vi "GenWave.vi"(2 "Sampling Rate (MHz)":u32=1000, 3 "Start Gap":dbl, 4 "Start Time":dbl, 5 "Offset":dbl min=-1.0 max=1.0 step=0.1 format="%.2p", 6 "T0":dbl, 7 "Wave":T1 {"Phase (Pi)" min=-1.0 max=1.0 step=0.1 format="%.2f"; "Gap (us)" format="%.2f"; "Amplitude" format="%.2f"; "Duration (us)" format="%.2f"; "Frequency (MHz)" format="%.4f"}) -> (0 "End Time":dbl, 1 "Output":i16[](array[numeric]))   [LabVIEW 2014]
uses:
  Wave.ctl
  <vilib>/gmath/NI_Gmath.lvlib
panel:
  in  "Sample Length Unit":u32=32
  in  "Minimal Sample Length":i32=192
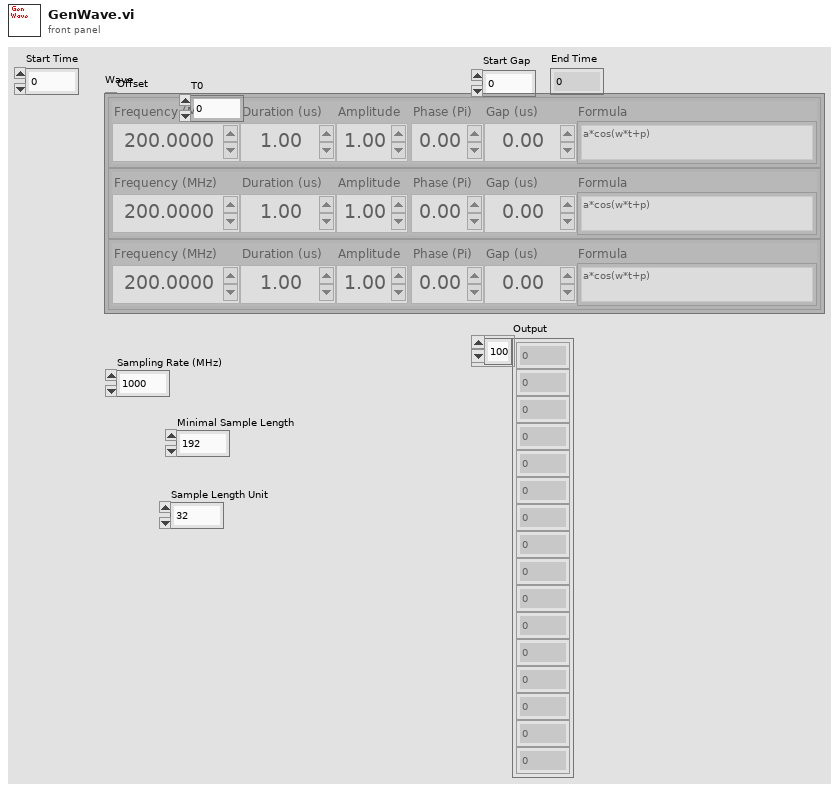
[diagram p1: front panel]
types:
  T1 = typedef "Wave.ctl" = cluster{"Frequency (MHz)":dbl, "Duration (us)":dbl, "Amplitude":dbl, "Phase (Pi)":dbl, "Gap (us)":dbl, "Formula":string}[]
  T2 = cluster{"parameter name":string, "parameter content":string}[]
  T3 = cluster{string, "formula after substitution":string}
  T4 = cluster{"Frequency (MHz)":dbl, "Duration (us)":dbl, "Amplitude":dbl, "Phase (Pi)":dbl, "Gap (us)":dbl, "Formula":string}
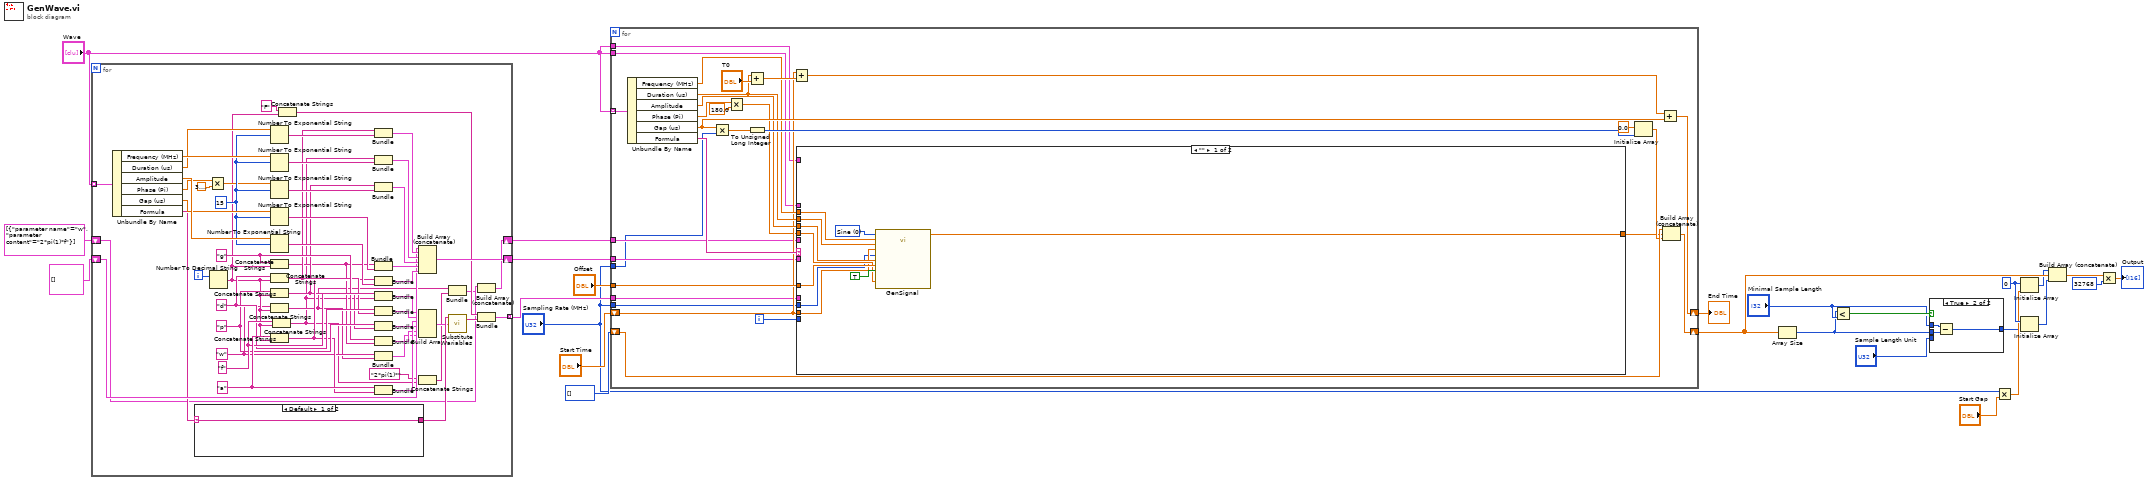
[diagram p0: block diagram]
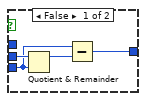
[diagram p2: hidden frame]
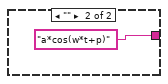
[diagram p3: hidden frame]
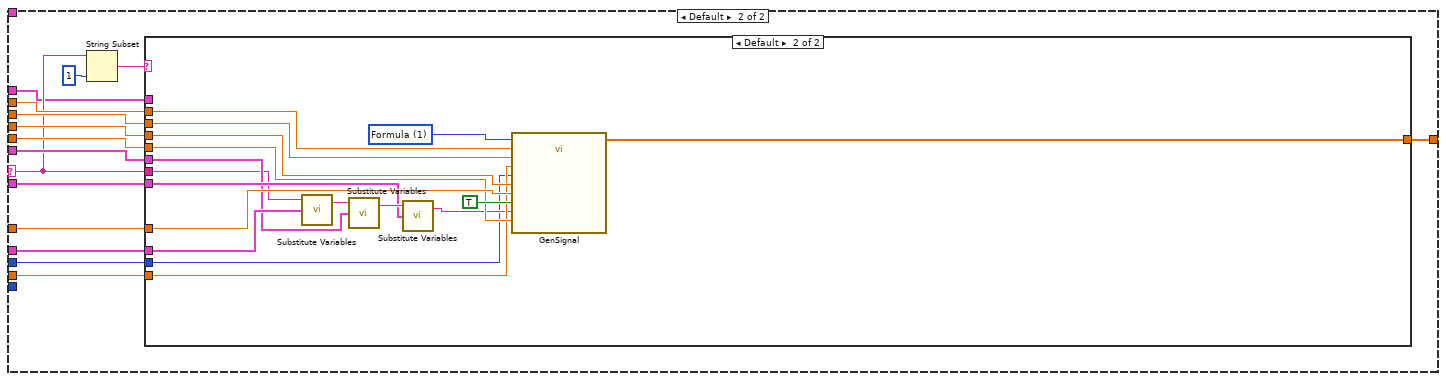
[diagram p4: hidden frame]
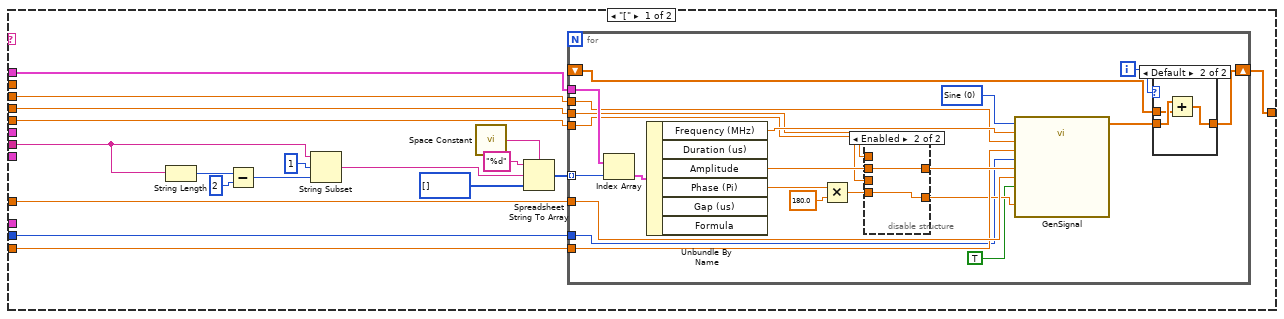
[diagram p5: hidden frame]
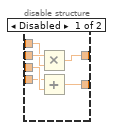
[diagram p6: hidden frame]
diagram:
  w14 = u32 0 ("element")
  n1 = for {
    tunnel: "Wave" -> [w62] mode=indexing
    shift-right: [w63] -> w19
    shift-left: cluster{string, string}[] [] -> [w64]
    tunnel: [w40] -> w18 mode=indexing
    shift-right: [w26] -> w15
    shift-left: T2 [{"parameter name"="w", "parameter content"="2*pi(1)*f"}] ("Substitution Rules") -> [w28]
    i -> [w65]
    w34 = "w" ("string")
    w69 = i16 15 ("width (-)")
    w56 = "a" ("string")
    w54 = "f" ("string")
    w43 = "g" ("string")
    w46 = "p" ("string")
    w50 = "d" ("string")
    n2 = Unbundle By Name(w62) -> ("Frequency (MHz)"=w78:dbl, "Duration (us)"=w77:dbl, "Amplitude"=w76:dbl, "Phase (Pi)"=w67:dbl, "Gap (us)"=w75:dbl, "Formula"=w59:string)
    n3 = case shown="Default" w59 {
      selector: w59 -> [w79 _]
      tunnel: [w79 "a*cos(w*t+p)"] -> w58
      frame Default {
      }
      frame "" {
      }
    }
    n4 = Multiply(x=w67, y=3.141592653589793) -> (x*y=w66:dbl)
    n5 = Number To Decimal String(number=w65) -> (decimal integer string=w35:string)  [unwired: 1 in]
    n6 = Number To Exponential String(number=w77, 3:w69) -> (E-format string=w49:string)  [unwired: 2 in]
    n7 = Number To Exponential String(number=w78, 3:w69) -> (E-format string=w53:string)  [unwired: 2 in]
    n8 = Number To Exponential String(number=w66, 3:w69) -> (E-format string=w45:string)  [unwired: 2 in]
    n9 = Number To Exponential String(number=w75, 3:w69) -> (E-format string=w42:string)  [unwired: 2 in]
    n10 = Number To Exponential String(number=w76, 3:w69) -> (E-format string=w52:string)  [unwired: 2 in]
    n11 = Concatenate Strings(w43, w35) -> (w36:string)
    n12 = Concatenate Strings(w50, w35) -> (w39:string)
    n13 = Concatenate Strings(w46, w35) -> (w37:string)
    n14 = Concatenate Strings(w34, w35) -> (w32:string)
    n15 = Concatenate Strings(w56, w35) -> (w38:string)
    n16 = Concatenate Strings(w54, w35) -> (w30:string)
    n17 = Concatenate Strings("F" ("string"), w35) -> (w61:string)
    n18 = Bundle(w39, w49) -> (w74:cluster{string, string})  [unwired: 1 in]
    n19 = Bundle(w30, w53) -> (w73:cluster{string, string})  [unwired: 1 in]
    n20 = Bundle(w37, w45) -> (w72:cluster{string, string})  [unwired: 1 in]
    n21 = Bundle(w36, w42) -> (w71:cluster{string, string})  [unwired: 1 in]
    n22 = Bundle(w38, w52) -> (w70:cluster{string, string})  [unwired: 1 in]
    n23 = Bundle("string"=w54, w30) -> (w48:cluster{"string":string, string})  [unwired: 1 in]
    n24 = Bundle("string"=w50, w39) -> (w47:cluster{"string":string, string})  [unwired: 1 in]
    n25 = Bundle("string"=w46, w37) -> (w44:cluster{"string":string, string})  [unwired: 1 in]
    n26 = Bundle("string"=w43, w36) -> (w41:cluster{"string":string, string})  [unwired: 1 in]
    n27 = Bundle("string"=w34, w32) -> (w33:cluster{"string":string, string})  [unwired: 1 in]
    n28 = Bundle("string"=w56, w38) -> (w55:cluster{"string":string, string})  [unwired: 1 in]
    n29 = Build Array (concatenate)(w64, w74, w73, w72, w71, w70) -> (w63:cluster{string, string}[])
    n30 = Build Array(w48, w47, w55, w44, w41, w33) -> (w51:cluster{"string":string, string}[])
    n31 = Concatenate Strings("2*pi(1)*" ("string"), w30) -> (w29:string)
    n32 = Bundle(w32, w29) -> (w27:cluster{string, string})  [unwired: 1 in]
    n33 = call <vilib>:"Substitute Variables.vi"("Substitution Rules"=w51, "original formula"=w58) -> ("formula after substitution"=w57:string)  [unwired: 1 in, 1 out]
    n34 = Build Array (concatenate)(w28, w27) -> (w26:T2)
    n35 = Bundle(w61, "formula after substitution"=w57) -> (w40:T3)  [unwired: 1 in]
  }
  n36 = for {
    tunnel: "Wave" -> [w99] mode=indexing
    shift-right: [w109] -> w20
    shift-left: "Start Time" -> [w90]
    tunnel: "Offset" -> [w95]
    shift-right: [w108] -> w21
    shift-left: u16[] [] -> [w107]
    tunnel: "Wave" -> [w89]
    tunnel: w19 -> [w87]
    tunnel: w18 -> [w86]
    tunnel: w15 -> [w85]
    tunnel: "Sampling Rate (MHz)" -> [w84]
    tunnel: "Sampling Rate (MHz)" -> [w83]
    tunnel: "Wave" -> [w82]
    i -> [w88]
    n37 = Unbundle By Name(w99) -> ("Frequency (MHz)"=w92:dbl, "Duration (us)"=w96:dbl, "Amplitude"=w97:dbl, "Phase (Pi)"=w91:dbl, "Gap (us)"=w105:dbl, "Formula"=w94:string)
    n38 = Multiply(x=w105, y=w84) -> (x*y=w102:dbl)
    n39 = Multiply(x=w91, y=180.0) -> (x*y=w81:dbl)
    n40 = Add(x=w96, y="T0") -> (x+y=w104:dbl)
    n41 = To Unsigned Long Integer(number=w102) -> (unsigned 32bit integer=w100:u32)
    n42 = Add(x=w90, y=w104) -> (x+y=w110:dbl)
    n43 = case shown="\"\"" w94 {
      selector: w94 -> [_ w122]
      tunnel: [w120 w131] -> w98
      tunnel: w92 -> [w111 w135]
      tunnel: w97 -> [w117 w133]
      tunnel: w96 -> [w116 w134]
      tunnel: w95 -> [w115 w132]
      tunnel: w81 -> [w114 w130]
      tunnel: w90 -> [w113 w129]
      tunnel: w89 -> [_ _]
      tunnel: w88 -> [_ _]
      tunnel: w87 -> [_ w128]
      tunnel: w86 -> [_ w127]
      tunnel: w85 -> [_ w126]
      tunnel: w83 -> [w112 w125]
      tunnel: w82 -> [_ w121]
      frame "" {
        w119 = u16 0 items=["Sine", "Formula"] ("Signal Type")
        n44 = call "GenSignal.vi"("Offset"=w115, "Reset Signal"=TRUE, "Amplitude"=w117, "Sampling Rate (MHz)"=w112, "Phase"=w114, "Start Time"=w113, "Duration (us)"=w116, "Frequency (MHz)"=w111, "Signal Type"=w119) -> ("Wave"=w120:dbl[])  [unwired: 1 in, 1 out]
      }
      frame Default {
        n45 = String Subset(string=w122, length (rest)=1 ("length (rest)")) -> (substring=w123:string)  [unwired: 1 in]
        n46 = case shown="Default" w123 {
          tunnel: w135 -> [_ w203]
          tunnel: w134 -> [w138 w202]
          tunnel: w133 -> [w142 w201]
          tunnel: w132 -> [w141 w200]
          tunnel: [w136 w198] -> w131
          tunnel: w130 -> [w139 w197]
          tunnel: w129 -> [w140 w196]
          tunnel: w128 -> [_ w193]
          tunnel: w127 -> [_ w192]
          tunnel: w126 -> [_ w190]
          tunnel: w125 -> [w137 w189]
          tunnel: w122 -> [w144 w188]
          tunnel: w121 -> [w143 _]
          frame "[" {
            n47 = String Length(string=w144) -> (length=w153:i32)
            n48 = Subtract(x=w153, y=2) -> (x-y=w151:i32)
            n49 = String Subset(string=w144, offset (0)=1, length (rest)=w151) -> (substring=w149:string)
            n50 = call <vilib>:"Space Constant.vi"() -> ("String"=w147:string)
            n51 = Spreadsheet String To Array(delimiter (Tab)=w147, format string="%d", spreadsheet string=w149, array type (2D Dbl)=i32[] []) -> (array=w145:i32[])
            n52 = for {
              tunnel: w145 -> [w174] mode=indexing
              tunnel: w143 -> [w175]
              tunnel: w142 -> [w170]
              tunnel: w141 -> [w168]
              tunnel: w140 -> [w167]
              tunnel: w138 -> [w164]
              tunnel: w139 -> [w163]
              tunnel: w137 -> [w162]
              shift-right: [w159] -> w136
              shift-left: _ -> [w158]
              i -> [w157]
              w161 = u16 0 items=["Sine", "Formula"] ("Signal Type")
              n53 = Index Array(array=w175, index=w174) -> (element=w173:T4)
              n54 = Unbundle By Name(w173) -> ("Frequency (MHz)"=w172:dbl, "Amplitude"=w171:dbl, "Phase (Pi)"=w155:dbl)  [unwired: 3 out]
              n55 = Multiply(x=w155, y=180.0) -> (x*y=w154:dbl)
              n56 = disable-structure shown="Enabled" {
                disable-tunnel: w171 -> [w181 w183]
                disable-tunnel: w170 -> [w180 _]
                disable-tunnel: [w179 w183] -> w169
                disable-tunnel: w154 -> [w176 w182]
                disable-tunnel: [w178 w182] -> w166
                disable-tunnel: w163 -> [w177 _]
                frame Disabled {
                  n57 = Multiply(x=w181, y=w180) -> (x*y=w179:dbl)
                  n58 = Add(x=w176, y=w177) -> (x+y=w178:dbl)
                }
                frame Enabled {
                }
              }
              n59 = call "GenSignal.vi"("Offset"=w168, "Reset Signal"=TRUE, "Amplitude"=w169, "Sampling Rate (MHz)"=w162, "Phase"=w166, "Start Time"=w167, "Duration (us)"=w164, "Frequency (MHz)"=w172, "Signal Type"=w161) -> ("Wave"=w160:dbl[])  [unwired: 1 in, 1 out]
              n60 = case shown="Default" w157 {
                tunnel: w160 -> [w184 w187]
                tunnel: [w184 w186] -> w159
                tunnel: w158 -> [_ w185]
                frame 0 {
                }
                frame Default {
                  n61 = Add(x=w187, y=w185) -> (x+y=w186:dbl[])
                }
              }
            }
          }
          frame Default {
            w204 = u16 1 items=["Sine", "Formula"] ("Signal Type")
            n62 = call <vilib>:"Substitute Variables.vi"("Substitution Rules"=w192, "original formula"=w188) -> ("formula after substitution"=w191:string)  [unwired: 1 in, 1 out]
            n63 = call <vilib>:"Substitute Variables.vi"("Substitution Rules"=w190, "original formula"=w191) -> ("formula after substitution"=w194:string)  [unwired: 1 in, 1 out]
            n64 = call <vilib>:"Substitute Variables.vi"("Substitution Rules"=w193, "original formula"=w194) -> ("formula after substitution"=w195:string)  [unwired: 1 in, 1 out]
            n65 = call "GenSignal.vi"("Offset"=w200, "Reset Signal"=TRUE, "Formula"=w195, "Amplitude"=w201, "Sampling Rate (MHz)"=w189, "Phase"=w197, "Start Time"=w196, "Duration (us)"=w202, "Frequency (MHz)"=w203, "Signal Type"=w204) -> ("Wave"=w198:dbl[])  [unwired: 1 out]
          }
        }
      }
    }
    n66 = Initialize Array(0.0 ("element"), w100) -> (w101:dbl[])
    n67 = Add(x=w110, y=w105) -> (x+y=w109:dbl)
    n68 = Build Array (concatenate)(w107, w98, w101) -> (w108:dbl[])
  }
  "End Time" <- w20
  n69 = Array Size(array=w21) -> (size(s)=w8:i32)
  n70 = Less?(x=w8, y="Minimal Sample Length") -> (x < y?=w10:bool)
  n71 = case shown="True" w10 {
    tunnel: [w206 w209] -> w6
    tunnel: "Sample Length Unit" -> [w205 _]
    tunnel: "Minimal Sample Length" -> [_ w211]
    tunnel: w8 -> [w208 w210]
    frame False {
      n72 = Quotient & Remainder(x=w208, y=w205) -> (x-y*floor(x/y)=w207:u32)  [unwired: 1 out]
      n73 = Subtract(x=w205, y=w207) -> (x-y=w206:u32)
    }
    frame True {
      n74 = Subtract(x=w211, y=w210) -> (x-y=w209:i32)
    }
  }
  n75 = Multiply(x="Sampling Rate (MHz)", y="Start Gap") -> (x*y=w11:dbl)
  n76 = Initialize Array(w14, w11) -> (w13:u32[])
  n77 = Initialize Array(w14, w6) -> (w22:u32[])
  n78 = Build Array (concatenate)(w13, w21, w22) -> (w3:dbl[])
  n79 = Multiply(x=w3, y=32768) -> (x*y=→"Output":dbl[])
